vi "Actor Core.vi"(8 "error in":errorcluster, 11 "Service Config Display in":refnum<class "Service Config Display.lvclass">) -> (0 "error out":errorcluster, 3 "Actor out":refnum<class "Actor.lvclass">)   [LabVIEW 2016, in "Assert API Components.lvlib" / "Assert Display.lvlib" / "Service Config Display.lvlib" / "Service Config Display.lvclass"]
doc: "(<B>Filename</B>: Actor Framework.lvlib:Actor.lvclass:Actor Core.vi)\n\nReceives messages to the actor, reacts to them, and initiates any error handling that may shut the actor down.\n\nDescendant classes may override this VI to append parallel tasks for the actor to complete while it handles messages. Overrides use the Call Parent Method node."
uses:
  Service Config Display.lvclass
  C:/Program Files (x86)/National Instruments/LabVIEW 2016/vi.lib/ActorFramework/Actor/Actor.lvclass
  C:/Users/ukhornp/Documents/Projects/actor_assert_api/Core/Base UI Actor/Base UI Actor/Base UI Actor.lvclass
  C:/Users/ukhornp/Documents/Projects/actor_assert_api/Core/Base UI Component/Base UI Component/Base UI Component.lvclass
  <vilib>/ActorFramework/Actor/Actor.lvclass
  Service Config Display.lvclass/Service Config Display.ctl
  Base UI Component/Base UI Component/Base UI Component.lvclass/Base UI Component.ctl
  Base UI Actor/Base UI Actor/Base UI Actor.lvclass/Base UI Actor.ctl
  <vilib>/ActorFramework/Actor/Actor.lvclass/Actor.ctl
  <vilib>/ActorFramework/Message Enqueuer/Message Enqueuer.lvclass/Message Enqueuer.ctl
  <vilib>/ActorFramework/Message Enqueuer/Init from Existing Queue.vi
  Base UI Component/Base UI Component/Base UI Component.lvclass
  <vilib>/ActorFramework/Message Enqueuer/Message Enqueuer.lvclass
  Base UI Actor/Base UI Actor/Base UI Actor.lvclass
panel:
  in  "Services":i32(listbox)
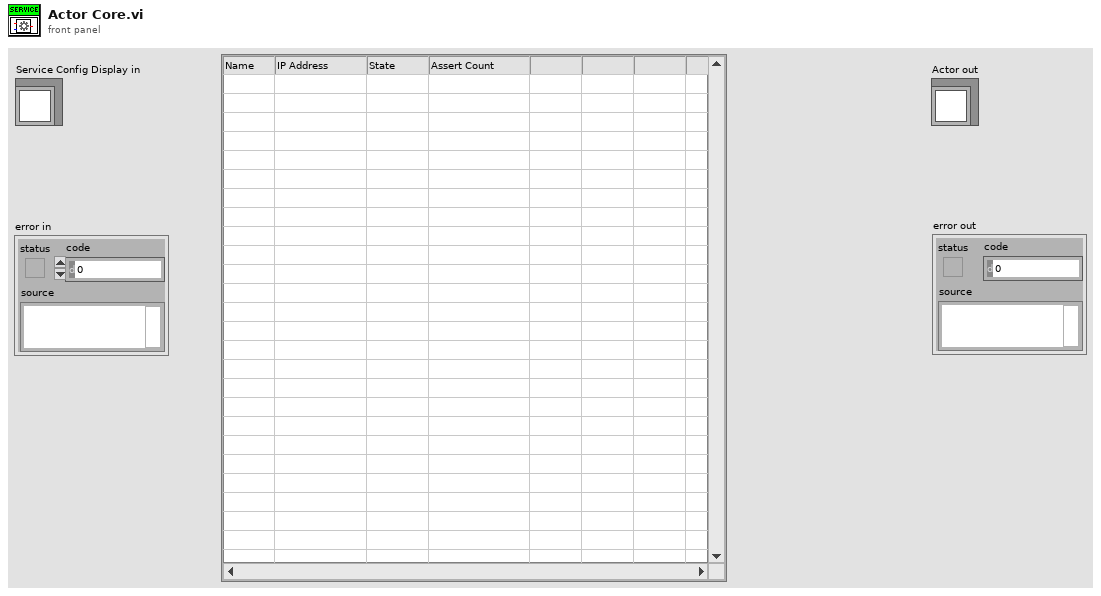
[diagram p1: front panel]
types:
  T1 = typedef "LVPoint32TypeDef.ctl" = cluster{"Horizontal":i32, "Vertical":i32}
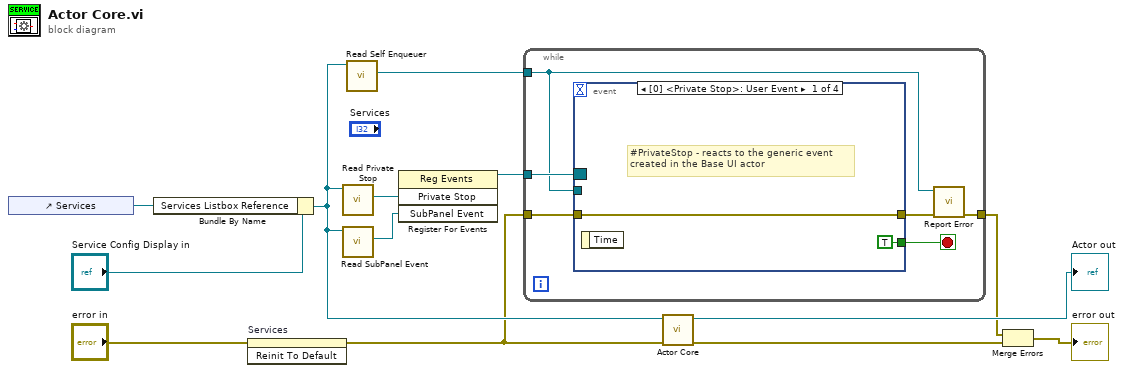
[diagram p0: block diagram]
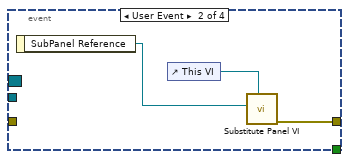
[diagram p2: hidden frame]
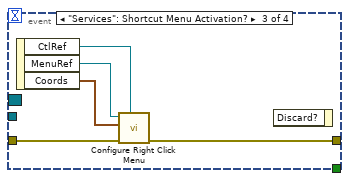
[diagram p3: hidden frame]
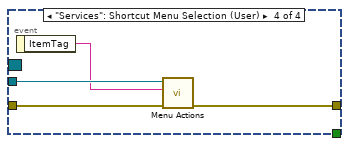
[diagram p4: hidden frame]
diagram:
  n1 = control-ref of="Services"() -> (w2:refnum<vi>)
  n2 = Bundle By Name(cluster="Service Config Display in", "Services Listbox Reference"=w2) -> (w3:refnum<class "Service Config Display.lvclass">)
  n3 = invoke on="Services" class="MCListbox (strict)" method="Reinit To Default"(error in="error in") -> (error out=w1:errorcluster)  [unwired: 2 in, 2 out]
  n4 = call "Read Private Stop.vi"("Base UI Actor in"=w3) -> ("Private Stop"=w11:refnum<user-event>)  [unwired: 10 in]
  n5 = call "Read SubPanel Event.vi"("Base UI Component in"=w3) -> ("SubPanel Event"=w10:refnum<user-event>)  [unwired: 10 in]
  n6 = call <vilib>:"Read Self Enqueuer.vi"("Actor"=w3) -> ("Self Enqueuer"=w5:refnum<class "Message Enqueuer.lvclass">)  [unwired: 10 in]
  n7 = register-events(w11, w10) -> (reference out=w9:refnum<event-registration>)  [unwired: 2 in, 1 out]
  n8 = while {
    tunnel: w9 -> [w19]
    tunnel: [w16] -> w7
    tunnel: w5 -> [w14]
    tunnel: w1 -> [w15]
    stop <- w17 stop-if-true
    n9 = event shown="[0] <Private Stop>: User Event" {
      selector: w19 -> [_ _ _ _]
      dyn-events: _ -> [_ _ _ _]
      timeout: _ -> [_ _ _ _]
      tunnel: [w20 w24 w28 w31] -> w18
      tunnel: [TRUE _ _ _] -> w17
      tunnel: w15 -> [w20 _ w27 w32]
      tunnel: w14 -> [_ _ _ w33]
      event User Event {
        # "#PrivateStop - reacts to the generic event created in the Base UI actor"
        n10 = event-data() -> ()  [unwired: 1 in, 1 out]
      }
      event User Event {
        n11 = event-data() -> ("SubPanel Reference"=w23:refnum<vi>)  [unwired: 1 in]
        n12 = control-ref of="This VI"() -> (w22:refnum<vi>)
        n13 = call "Substitute Panel VI.vi"("VI Reference"=w22, "SubPanel Reference"=w23) -> ("error out"=w24:errorcluster)  [unwired: 9 in]
      }
      event "Services": Shortcut Menu Activation? {
        n14 = event-data() -> ("CtlRef"=w25:refnum<vi>, "MenuRef"=w29:refnum<k9>, "Coords"=w26:T1)  [unwired: 1 in]
        n15 = call "Configure Right Click Menu.vi"("Table Reference"=w25, "error in (no error)"=w27, "Point32"=w26, "Menu in"=w29) -> ("error out"=w28:errorcluster)  [unwired: 7 in]
        n16 = event-data() -> ()  [unwired: 2 in, 1 out]
      }
      event "Services": Shortcut Menu Selection (User) {
        n17 = event-data() -> ("ItemTag"=w30:string)  [unwired: 1 in]
        n18 = call "Menu Actions.vi"("error in (no error)"=w32, "Tag"=w30, "Self Enqueuer"=w33) -> ("error out"=w31:errorcluster)  [unwired: 8 in]
      }
    }
    n19 = call "Report Error.vi"("error in (no error)"=w18, "Self Enqueuer"=w14) -> ("error out"=w16:errorcluster)  [unwired: 9 in]
  }
  n20 = call-parent "Actor Core.vi"("error in"=w1, "Actor in"=w3) -> ("error out"=w13:errorcluster, "Actor out"=→"Actor out":refnum<class "Actor.lvclass">)  [unwired: 8 in]
  n21 = Merge Errors(w7, w13) -> (→"error out":errorcluster)
